vi "Close Instrument Sessions.vi"(0 "Vector Abstract Path Group in":refnum<class "Vector Abstract Path Group.lvclass">, 11 "error in (no error)":errorcluster) -> (4 "Vector Abstract Path Group out":refnum<class "Vector Abstract Path Group.lvclass">, 15 "error out":errorcluster)   [LabVIEW 2023, in "RFFixtureCharact.Public.lvlib" / "Vector Abstract Path Group.lvclass"]
uses:
  Vector Abstract Path Group.lvclass
  Vector Abstract Path Group.lvclass/Vector Abstract Path Group.ctl
  Instruments/Cal Standard/Cal Standard Factory/Cal Standard Factory.lvclass
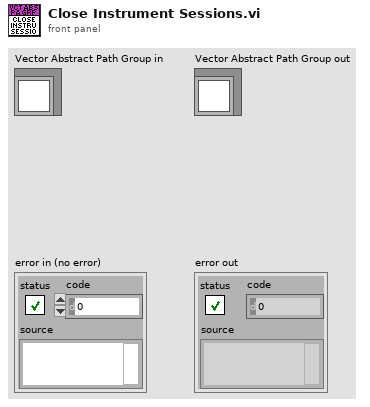
[diagram p1: front panel]
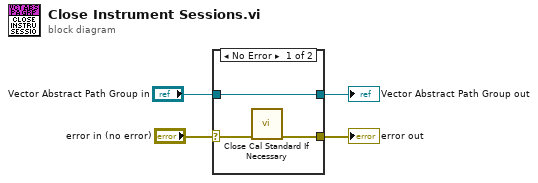
[diagram p0: block diagram]
diagram:
  n1 = case shown="No Error" "error in (no error)" {
    selector: "error in (no error)" -> [w6 w9]
    tunnel: [w5 w9] -> w1
    tunnel: [w7 w8] -> w2
    tunnel: "Vector Abstract Path Group in" -> [w7 w8]
    frame No Error {
      n2 = call "Close Cal Standard If Necessary.vi"("error in (no error)"=w6) -> ("error out"=w5:errorcluster)  [unwired: 14 in]
    }
    frame Error {
    }
  }
  "error out" <- w1
  "Vector Abstract Path Group out" <- w2
